vi "Dice simulation.vi"() -> ()   [LabVIEW 2024]
uses:
  <vilib>/numeric/Random Number (Range) U64.vi
  <vilib>/numeric/sub_Random U32.vi
panel:
  out "Time counter (sec.)":dbl
  out "Iteration counter":i32
  out "?":bool
  in  "Number of times in a row":dbl
  in  "Value":dbl min=1.0 max=6.0
  out "Dice throw result":u64[](array[numeric])
  in  "stop":bool
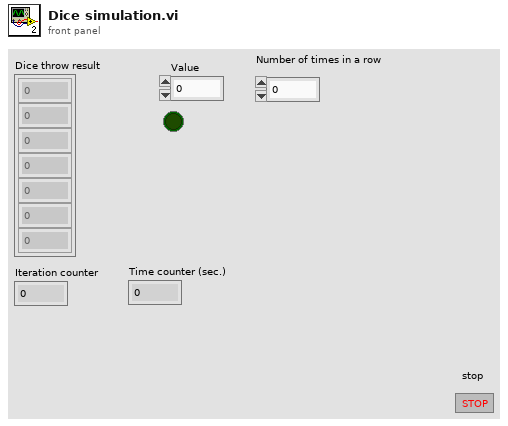
[diagram p1: front panel]
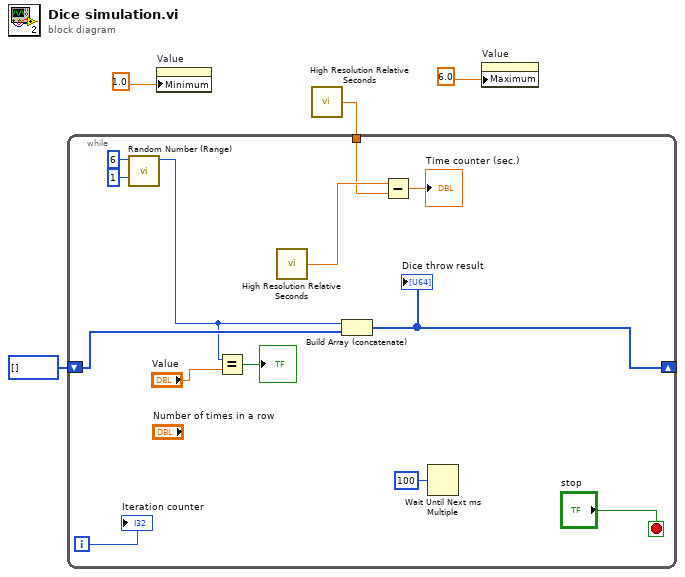
[diagram p0: block diagram]
diagram:
  n1 = property on="Value" class="DigNum (strict)"("Minimum"=1.0 ("Data Entry Limits:Minimum")) -> ()  [unwired: 2 in, 2 out]
  n2 = call <vilib>:"High Resolution Relative Seconds.vi"() -> ("relative seconds"=w2:dbl)
  n3 = while {
    shift-right: [w15] -> _
    shift-left: u64[] [] -> [w14]
    tunnel: w2 -> [w6]
    i -> [w9]
    stop <- "stop" stop-if-true
    n4 = call-poly <vilib>:"Random Number (Range).vi"("lower bound (0)"=u64 1, "upper bound (100)"=u64 6) -> ("number"=w12:u64)  [unwired: 9 in]
    n5 = Equal?(x=w12, y="Value") -> (x = y?=→"?":bool)
    n6 = call <vilib>:"High Resolution Relative Seconds.vi"() -> ("relative seconds"=w7:dbl)
    n7 = Build Array (concatenate)(w12, w14) -> (w15:u64[])
    "Dice throw result" <- w15
    n8 = Subtract(x=w7, y=w6) -> (x-y=→"Time counter (sec.)":dbl)
    n9 = Wait Until Next ms Multiple(millisecond multiple=u32 100) -> ()  [unwired: 1 out]
    "Iteration counter" <- w9
  }
  n10 = property on="Value" class="DigNum (strict)"("Maximum"=6.0 ("Data Entry Limits:Maximum")) -> ()  [unwired: 2 in, 2 out]
